vi "main_test.vi"() -> ()   [LabVIEW 2018]
uses:
  <vilib>/addons/database/Connection.llb/DB Tools Open Connec (Path).vi
  <vilib>/addons/database/NI_Database_API.lvlib
panel:
  out "时间":timestamp format="%<%H:%M:%S\n%Y/%m/%d>T"
  out "负责人数据":T1
  out "数据采集":bool=TRUE
  out "flaginit":bool=TRUE
  in  "下限":sgl=2.0 format="%#.2g"
  in  "上限":sgl=12.0 format="%#.2g"
  out "温度报警":string[][](table)
  out "疫苗信息":string[][](table)
  out "uid":i16
  out "途径地点":i32
  out "运输路径":cluster{"city":string, "布尔":T2}[](array[cluster])
  out "error out":errorcluster
  out "负责人信息":T1
  in  "YSJJ":bool
  out "定位":bool
  out "温度":sgl(graph)
  out "纬度":string
  out "经度":string
  in  "地图比例":i8(slide)=10 scale=6.0..18.0
  in  "地图":refnum<k7>(container) caption="网页浏览器"
  in  "Setvi":bool
  in  "停止":bool
  # "疫苗冷链储运监控系统\nVACCINE COLD-CHAIN TRANSPORTATION MONITORING SYSTEM"
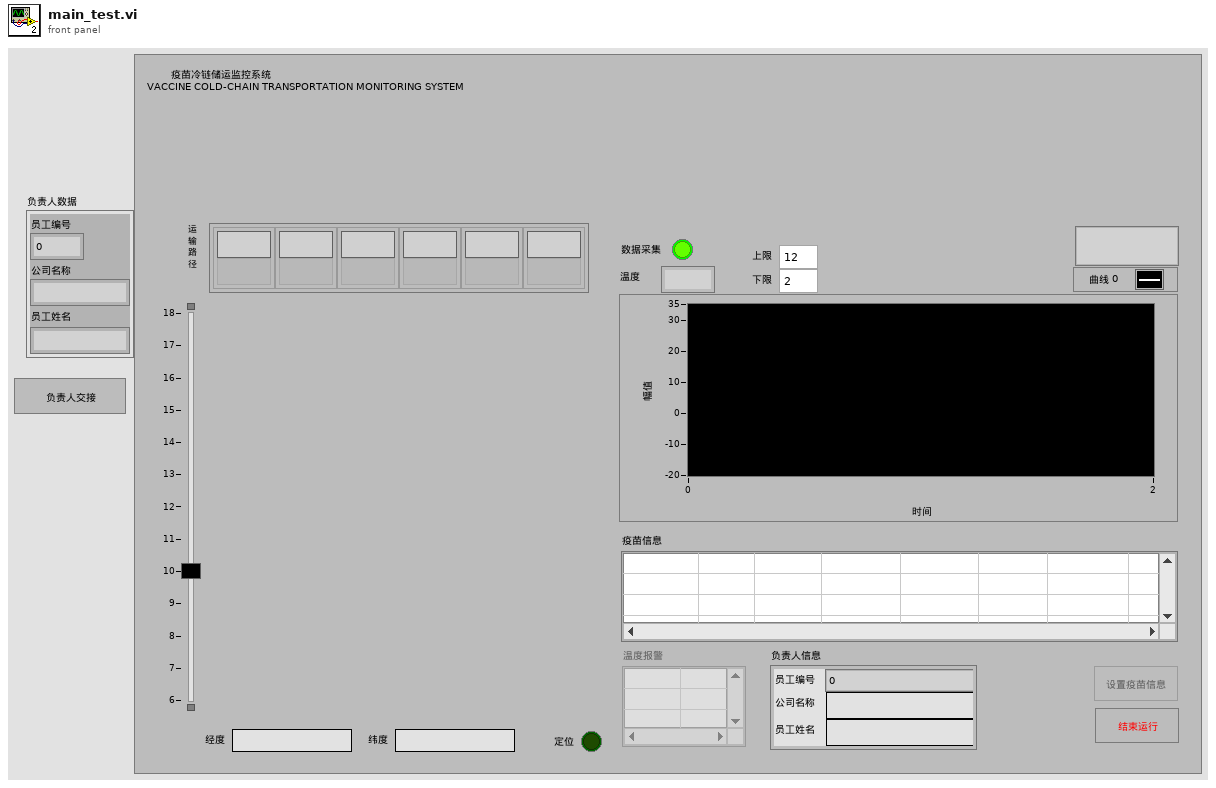
[diagram p1: front panel]
types:
  T1 = typedef "人员信息.ctl" = cluster{"员工编号":i32, "公司名称":string, "员工姓名":string}
  T2 = typedef "car.ctl" = bool
  T3 = enum8{"Enabled", "Disabled", "Disabled and Grayed Out"}
  T4 = typedef "NI_Database_API.lvlib/Conn ObjectReference.ctl" = refnum<k1>
  T5 = typedef "储运信息.ctl" = cluster{"纬度":sgl, "经度":sgl, "温度":sgl, "负责人":i32, "区域":string, "记录时间":timestamp}
  T6 = typedef "疫苗信息.ctl" = cluster{"疫苗名":string, "疫苗编号":i32, "疫苗类型":string, "生产厂家":string, "生产日期":timestamp, "生产地":string, "生产负责人":string, "是否合格":string, "疫苗功能":string}
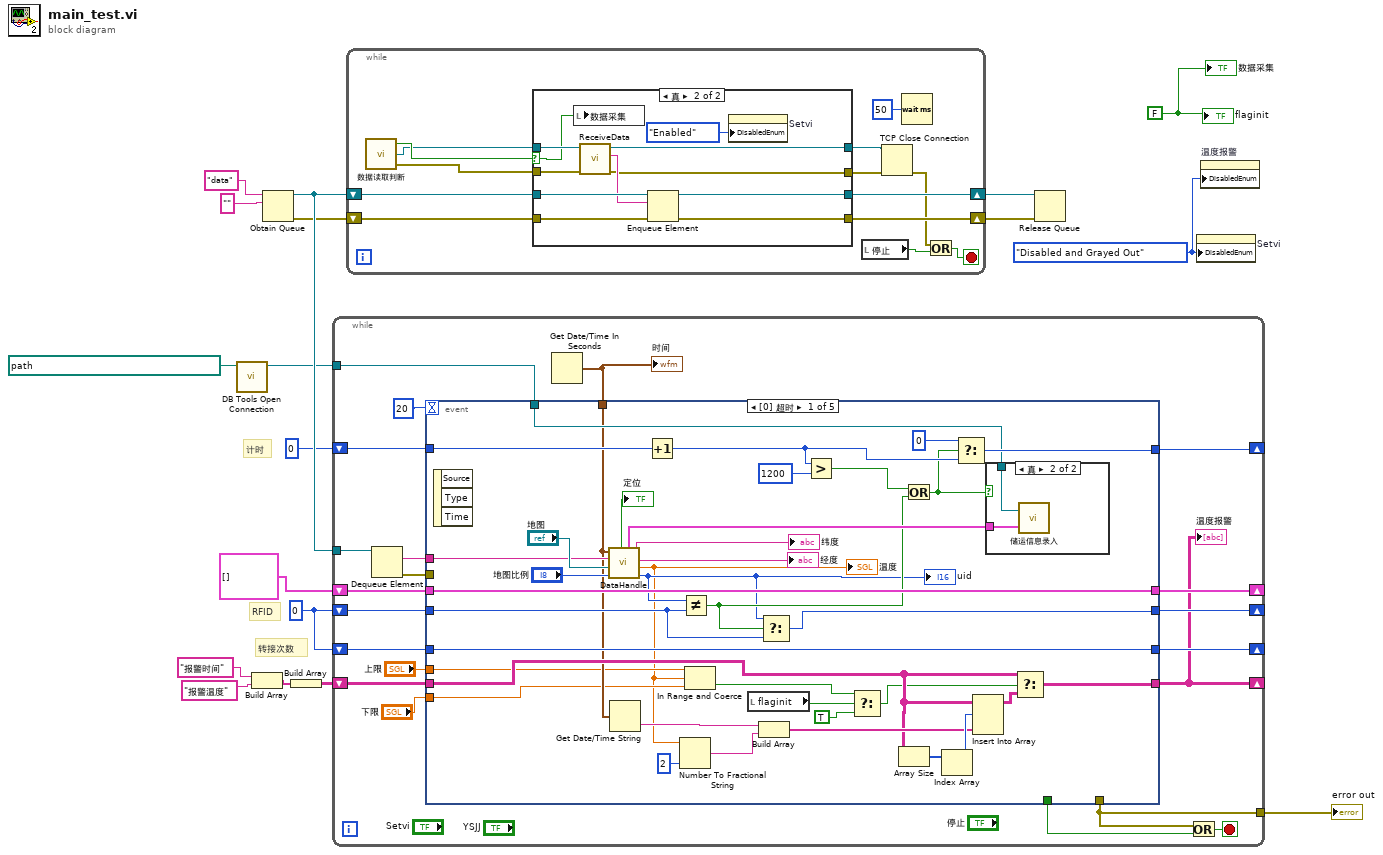
[diagram p0: block diagram]
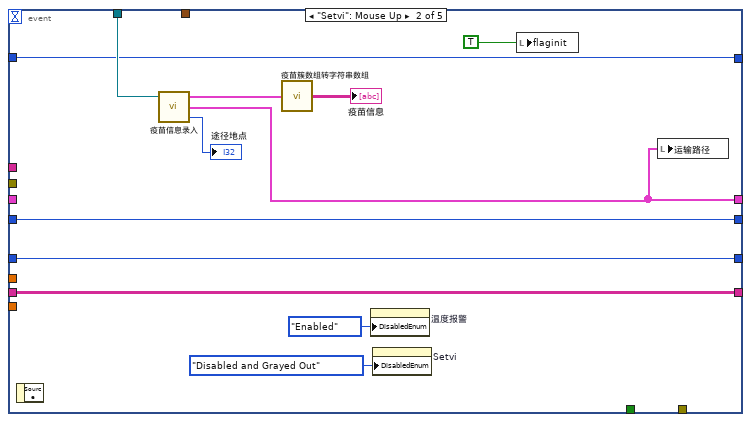
[diagram p3: hidden frame]
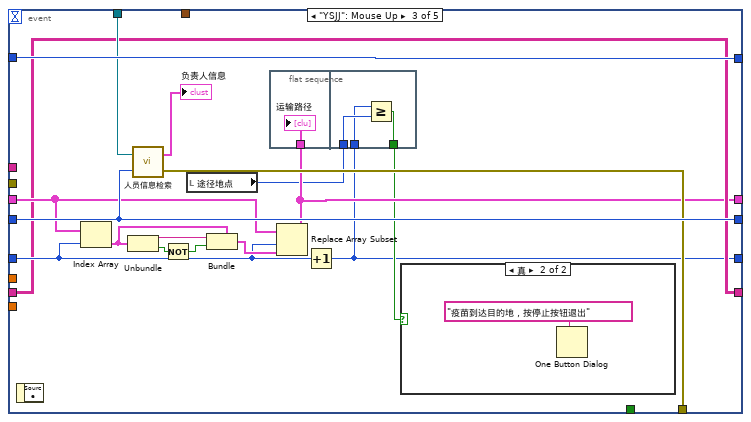
[diagram p4: hidden frame]
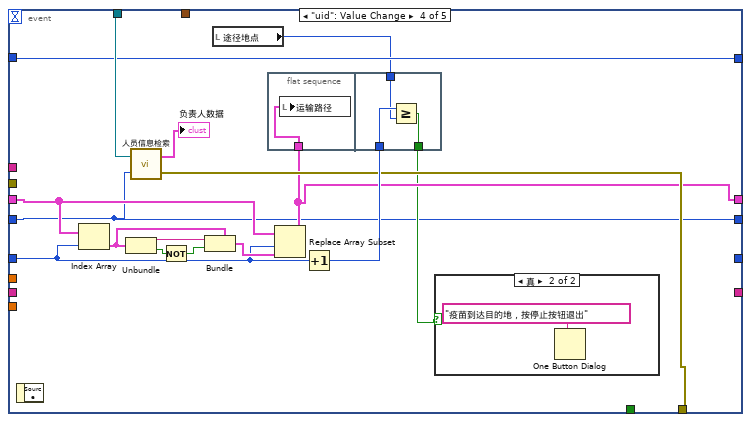
[diagram p6: hidden frame]
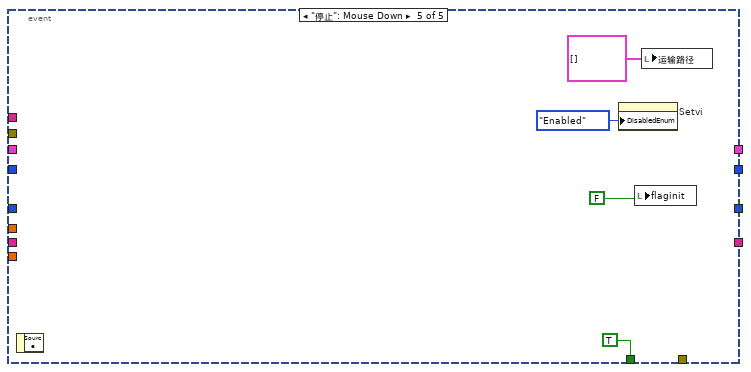
[diagram p8: hidden frame]
diagram:
  w2 = T3."Disabled and Grayed Out" ("禁用")
  w1 = FALSE
  w8 = 0
  # "转接次数"
  # "RFID"
  # "计时"
  n1 = call-poly <vilib>:"DB Tools Open Connection.vi"("connection information"=path "D:/2019毕业设计/Code/GPData.udl" ("路径")) -> ("connection reference"=w11:T4)  [unwired: 7 in, 1 out]
  n2 = Build Array("报警时间", "报警温度") -> (w5:string[])
  n3 = Obtain Queue(name (unnamed)="data" ("名称（未命名）"), element data type="" ("dataOut")) -> (queue out=w18:refnum<queue>, error out=w15:errorcluster)  [unwired: 3 in, 1 out]
  n4 = Build Array(w5) -> (w4:string[][])
  n5 = while {
    tunnel: w18 -> [w36]
    tunnel: w11 -> [w39]
    shift-right: [w34] -> _
    shift-left: 0 -> [w33]
    shift-right: [w32] -> _
    shift-left: w8 -> [w31]
    tunnel: [w28] -> w9
    shift-right: [w26] -> _
    shift-left: w8 -> [w25]
    shift-right: [w23] -> _
    shift-left: cluster{string, bool}[] [] -> [w24]
    shift-right: [w19] -> _
    shift-left: w4 -> [w20]
    stop <- w29 stop-if-true
    n6 = Dequeue Element(queue=w36) -> (element=w35:string, error out=w27:errorcluster)  [unwired: 2 in, 2 out]
    n7 = Get Date/Time In Seconds() -> (seconds since 1Jan1904=w37:timestamp)
    "时间" <- w37
    n8 = event shown="[0] 超时" {
      selector: _ -> [_ _ _ _ _]
      dyn-events: _ -> [_ _ _ _ _]
      timeout: 20 -> [_ _ _ _ _]
      tunnel: w39 -> [w65 w91 w107 w122 _]
      tunnel: [_ _ _ _ TRUE] -> w30
      tunnel: w37 -> [w44 _ _ _ _]
      tunnel: w35 -> [w72 _ _ _ _]
      tunnel: [w68 w90 w108 w121 _] -> w34
      tunnel: w33 -> [w71 w90 w108 w121 _]
      tunnel: [w59 w89 w105 w117 _] -> w32
      tunnel: w31 -> [w62 w89 w105 w117 _]
      tunnel: [_ _ w104 w123 _] -> w28
      tunnel: w27 -> [_ _ _ _ _]
      tunnel: [w64 w87 w92 _ _] -> w26
      tunnel: w25 -> [w64 w87 w97 w116 _]
      tunnel: [w63 w86 w95 w120 _] -> w23
      tunnel: w24 -> [w63 _ w99 w118 _]
      tunnel: "上限" -> [w42 _ _ _ _]
      tunnel: "下限" -> [w41 _ _ _ _]
      tunnel: w20 -> [w50 w82 w96 _ _]
      tunnel: [w57 w82 w96 _ _] -> w19
      event Timeout {
        n9 = event-data() -> ()  [unwired: 1 in, 3 out]
        n10 = call "DataHandle.vi"("滑动杆"="地图比例", "地图"="地图", "data"=w72, "时间"=w44) -> ("uid"=w45:i16, "温度"=w40:sgl, "经度显示"=→"经度":string, "纬度显示"=→"纬度":string, "储运信息簇"=w66:T5, "定位"=→"定位":bool)  [unwired: 1 in, 1 out]
        "温度" <- w40
        "uid" <- w45
        n11 = Get Date/Time String(seconds (now)=w44) -> (time string=w43:string)  [unwired: 2 in, 1 out]
        n12 = Increment(x=w71) -> (x+1=w69:i32)
        n13 = Number To Fractional String(number=w40, precision (6)=i16 2 ("精度(6)")) -> (F-format string=w53:string)  [unwired: 2 in]
        n14 = Not Equal?(x=w45, y=w62) -> (x != y?=w60:bool)
        n15 = In Range and Coerce(upper limit=w42, x=w40, lower limit=w41) -> (In Range?=w48:bool)  [unwired: 1 out]
        n16 = local read "flaginit"() -> (w49:bool)
        n17 = Build Array(w43, w53) -> (w52:string[])
        n18 = Select(t=w45, s=w60, f=w62) -> (s? t:f=w59:i32)
        n19 = Greater?(x=w69, y=1200) -> (0:w61:bool)
        n20 = Select(t=w48, s=w49, f=TRUE) -> (s? t:f=w46:bool)
        n21 = Array Size(array=w50) -> (size(s)=w56:i32[])
        n22 = Or(x=w61, y=w60) -> (x .or. y?=w58:bool)
        n23 = Index Array(array=w56) -> (element=w55:i32)  [unwired: 1 in]
        n24 = Select(t=0, s=w58, f=w69) -> (s? t:f=w68:i32)
        n25 = Insert Into Array(array=w50, index (row)=w55, new element=w52) -> (w51:string[][])  [unwired: 1 in]
        n26 = case shown="真" w58 {
          tunnel: w66 -> [_ w79]
          tunnel: w65 -> [_ w78]
          frame False {
          }
          frame True {
            n27 = call "储运信息录入.vi"("簇"=w79, "connection reference"=w78) -> ()  [unwired: 1 out]
          }
        }
        n28 = Select(t=w50, s=w46, f=w51) -> (s? t:f=w57:string[][])
      }
      event "Setvi": Mouse Up {
        n29 = event-data() -> ()  [unwired: 1 in, 1 out]
        n30 = call "疫苗信息录入.vi"("connection"=w91) -> ("途径地点"=→"途径地点":i32, "运输路线"=w86:cluster{"城市":string, bool}[], "疫苗信息"=w85:T6[])  [unwired: 2 in]
        n31 = call "疫苗簇数组转字符串数组.vi"("疫苗信息"=w85) -> ("疫苗信息"=→"疫苗信息":string[][])
        n32 = property on="温度报警" class="Tbl (严格)"("DisabledEnum"=T3."Enabled" ("禁用")) -> ()  [unwired: 2 in, 2 out]
        n33 = property on="Setvi" class="Bool (严格)"("DisabledEnum"=T3."Disabled and Grayed Out" ("禁用")) -> ()  [unwired: 2 in, 2 out]
        n34 = local write "flaginit"(TRUE) -> ()
        n35 = local write "运输路径"(w86) -> ()
      }
      event "YSJJ": Mouse Up {
        n36 = event-data() -> ()  [unwired: 1 in, 1 out]
        n37 = Index Array(array=w99, index=w97) -> (element=w100:cluster{string, bool})
        n38 = Unbundle(w100) -> (w101:string, w103:bool)
        n39 = call "人员信息检索.vi"("工作人员编号"=w105, "connection reference"=w107) -> ("error out"=w104:errorcluster, "负责人数据"=→"负责人信息":T1)
        n40 = Not(x=w103) -> (.not. x?=w102:bool)
        n41 = local read "途径地点"() -> (w94:i32)
        n42 = Bundle(cluster=w100, w101, w102) -> (w98:cluster{string, bool})
        n43 = flat-sequence {
          tunnel: w95 -> [w109]
          tunnel: w94 -> [w112]
          tunnel: [w111] -> w93
          tunnel: w92 -> [w110]
          frame #0 {
            "运输路径" <- w109
          }
          frame #1 {
            n44 = Greater Or Equal?(x=w110, y=w112) -> (x >= y?=w111:bool)
          }
        }
        n45 = Replace Array Subset(array=w99, new element=w98, index=w97) -> (w95:cluster{string, bool}[])
        n46 = Increment(x=w97) -> (x+1=w92:i32)
        n47 = case shown="真" w93 {
          frame False {
          }
          frame True {
            n48 = One Button Dialog(message="疫苗到达目的地，按停止按钮退出" ("消息")) -> ()  [unwired: 1 in, 1 out]
          }
        }
      }
      event "uid": Value Change {
        n49 = event-data() -> ()  [unwired: 1 in, 1 out]
        n50 = Index Array(array=w118, index=w116) -> (element=w126:cluster{string, bool})
        n51 = Unbundle(w126) -> (w127:string, w129:bool)
        n52 = call "人员信息检索.vi"("工作人员编号"=w117, "connection reference"=w122) -> ("error out"=w123:errorcluster, "负责人数据"=→"负责人数据":T1)
        n53 = Not(x=w129) -> (.not. x?=w128:bool)
        n54 = Bundle(cluster=w126, w127, w128) -> (w125:cluster{string, bool})
        n55 = local read "途径地点"() -> (w114:i32)
        n56 = flat-sequence {
          tunnel: w120 -> [w131]
          tunnel: [w134] -> w119
          tunnel: w124 -> [w133]
          tunnel: w114 -> [w132]
          frame #0 {
            n57 = local write "运输路径"(w131) -> ()
          }
          frame #1 {
            n58 = Greater Or Equal?(x=w133, y=w132) -> (x >= y?=w134:bool)
          }
        }
        n59 = Replace Array Subset(array=w118, new element=w125, index=w116) -> (w120:cluster{string, bool}[])
        n60 = Increment(x=w116) -> (x+1=w124:i32)
        n61 = case shown="真" w119 {
          frame False {
          }
          frame True {
            n62 = One Button Dialog(message="疫苗到达目的地，按停止按钮退出" ("消息")) -> ()  [unwired: 1 in, 1 out]
          }
        }
      }
      event "停止": Mouse Down {
        n63 = event-data() -> ()  [unwired: 1 in, 1 out]
        n64 = property on="Setvi" class="Bool (严格)"("DisabledEnum"=T3."Enabled" ("禁用")) -> ()  [unwired: 2 in, 2 out]
        n65 = local write "flaginit"(FALSE) -> ()
        n66 = local write "运输路径"(cluster{string, bool}[] []) -> ()
      }
    }
    "温度报警" <- w19
    n67 = Or(x=w28, y=w30) -> (x .or. y?=w29:bool)
  }
  "error out" <- w9
  n68 = while {
    shift-right: [w149] -> w14
    shift-left: w18 -> [w151]
    shift-right: [w148] -> w13
    shift-left: w15 -> [w150]
    stop <- w139 stop-if-true
    n69 = call "数据读取判断.vi"() -> ("error out"=w143:errorcluster, "connection ID"=w145:refnum<k5>, "判断错误"=w146:bool)
    n70 = case shown="真" w146 {
      selector: w146 -> [_ w156]
      tunnel: w151 -> [w155 w166]
      tunnel: w150 -> [w154 w165]
      tunnel: [w154 w164] -> w148
      tunnel: [w155 w163] -> w149
      tunnel: w145 -> [w153 w161]
      tunnel: [w153 w160] -> w144
      tunnel: w143 -> [w152 w159]
      tunnel: [w152 w158] -> w142
      frame False {
      }
      frame True {
        n71 = local write "数据采集"(w156) -> ()
        n72 = call "ReceiveData.vi"("错误输入（无错误）"=w159, "连接ID"=w161) -> ("错误输出"=w158:errorcluster, "dataOut"=w162:string, "连接ID输出"=w160:refnum<k5>)  [unwired: 5 in, 2 out]
        n73 = Enqueue Element(queue=w166, element=w162, error in (no error)=w165) -> (queue out=w163:refnum<queue>, error out=w164:errorcluster)  [unwired: 1 in, 1 out]
        n74 = property on="Setvi" class="Bool (严格)"("DisabledEnum"=T3."Enabled" ("禁用")) -> ()  [unwired: 2 in, 2 out]
      }
    }
    n75 = local read "停止"() -> (w140:bool)
    n76 = TCP Close Connection(connection ID=w144, error in (no error)=w142) -> (error out=w141:errorcluster)  [unwired: 1 in, 1 out]
    n77 = Wait (ms)(milliseconds to wait=u32 50 ("等待时间（毫秒）")) -> ()  [unwired: 1 out]
    n78 = Or(x=w141, y=w140) -> (x .or. y?=w139:bool)
  }
  n79 = Release Queue(queue=w14, error in (no error)=w13) -> ()  [unwired: 1 in, 3 out]
  n80 = property on="Setvi" class="Bool (严格)"("DisabledEnum"=w2) -> ()  [unwired: 2 in, 2 out]
  n81 = property on="温度报警" class="Tbl (严格)"("DisabledEnum"=w2) -> ()  [unwired: 2 in, 2 out]
  "flaginit" <- w1
  "数据采集" <- w1
